vi "Lockin-4461_Multiple Inputs and Outputs_KH_functional_global_waveform_generalized_f_parallel_exec.vi"(8 "stop":bool) -> ()   [LabVIEW 2013]
uses:
  <vilib>/Analysis/baseanly.llb/Mean (DBL).vi
  <vilib>/Analysis/2dsp.llb/Decimate (single shot).vi
  <vilib>/Analysis/2dsp.llb/Decimate (single shot, DBL).vi
  DAQ-Lockin-SubVI/Lock-in Globles Multiple Inputs and Outputs used with FGV.vi
  <vilib>/Utility/error.llb/Error Cluster From Error Code.vi
  <vilib>/Analysis/NI_AALBase.lvlib
panel:
  in  "X input signal":i8(slide) scale=1.0..8.0
  in  "X Tab Control 3":enum32{"Page 1", "Page 2"}(tab)
  in  "X zero offset 2":bool
  in  "X Enum":enum16{"X and Y", "R and Theta"}(ring)
  in  "X Cluster 2":T1
  in  "X AI Block Size":dbl
  in  "X order":dbl
  in  "X AI Buffer Size":dbl
  in  "X Boolean":bool
  in  "Input Signals":i16(slide)=1 scale=1.0..20.0
  out "phase log":dbl[](array[numeric])
  in  "Tab Control 2":T2(tab)=enum."Lock-in Settings"
  in  "AI Configuration":T3(array[cluster])=[{"AI.Coupling"=10050, "AI.Max"=10.0, "AI.Min"=-10.0, "Input physical channels"="PXI1Slot2/ai0:1"}, {"AI.Coupling"=10050, "AI.Max"=10.0, "AI.Min"=-10.0, "Input physical channels"="PXI1Slot3/ai0:1"}, {"AI.Coupling"=10050, "AI.Max"=10.0, "AI.Min"=-10.0, "Input physical channels"="PXI1Slot5/ai0:1"}, {"AI.Coupling"=10050, "AI.Max"=10.0, "AI.Min"=-10.0, "Input physical channels"="PXI1Slot6/ai0:1"}] {"AI.Coupling" items=["AC"=10045, "DC"=10050, "GND"=10066]}
  in  "AO Configuration":T4(array[cluster])=[{"Output physical channels"="PXI1Slot2/ao0:1", "AO. Max"=0.1, "AO.Min"=-0.1}, {"Output physical channels"="PXI1Slot3/ao0:1", "AO. Max"=0.25, "AO.Min"=-0.25}, {"Output physical channels"="PXI1Slot5/ao0:1", "AO. Max"=0.1, "AO.Min"=-0.1}, {"Output physical channels"="PXI1Slot6/ao0:1", "AO. Max"=0.1, "AO.Min"=-0.1}]
  in  "Lockin":T5={"REF f (Hz)"=[13.0, 13.0, 13.0, 13.0, 13.0, 13.0, 13.0, 13.0], "REF phi (deg)"=[0.0, 0.0, 0.0, 0.0, 0.0, 0.0, 0.0, 0.0]} {"REF phi (deg)" format="%#_3g"}
  in  "REF f = AO f?":bool
  in  "Gain":dbl[](array[numeric])=[1.0, 1.0, 1.0, 1.0, 1.0, 1.0, 1.0, 1.0]
  out "elapsed time":dbl=1410.416
  in  "zero offset":bool
  in  "measure offset":bool
  out "filter fC (Hz)":dbl=0.3183098861837907
  in  "TC (s)":dbl=0.5
  in  "order":i32=2
  in  "AO":T6={"AO amp (V)"=[0.1, 0.09, 0.08, 0.07, 0.06, 0.05, 0.04, 0.03], "AO DC (V)"=[0.0, 0.0, 0.0, 0.0, 0.0, 0.0, 0.0, 0.0], "AO f (Hz)"=[13.0, 13.0, 13.0, 13.0, 13.0, 13.0, 13.0, 13.0], "AO phi (deg)"=[0.0, 0.0, 0.0, 0.0, 0.0, 0.0, 0.0, 0.0], "function"=[enum."Sine Wave", enum."Sine Wave", enum."Sine Wave", enum."Sine Wave", enum."Sine Wave", enum."Sine Wave", enum."Sine Wave", enum."Sine Wave"]} {"AO DC (V)" format="%#_6p"; "AO amp (V)" format="%#_6p"}
  in  "all  f same?":bool
  in  "simulate?":bool=TRUE
  in  "reset signal":bool
  in  "AI Buffer Size (S)":i32=10
  in  "milliseconds to wait":u32=1000
  out "sampling info":cluster{"Fs":dbl, "#s":dbl}={"Fs"=204800.0, "#s"=15753.0}
  in  "pre filter fl":dbl=40.0
  in  "prefilter?":bool
  in  "reset REF phi to zero":bool
  in  "autophase?":bool
  in  "auto block size":bool=TRUE
  in  "P":dbl=0.5 format="%.2f"
  in  "I":dbl=0.6 format="%.2f"
  in  "D":dbl=0.019999999999999997 format="%.2f"
  out "Display 2":dbl=-0.01728566342801391 format="%.6p"
  out "Display 1":dbl=0.09985345527594 format="%.6p"
  in  "Display":enum16{"X and Y", "R and Theta"}(ring)=enum."R and Theta"
  out "AO Task":refnum<k21>[](array[refnum])
  out "AI task":refnum<k21>[](array[refnum])
  in  "Tab Control":T7(tab)
  out "Display X (or R)":waveform(dbl)[](graph)=[{"t0"=timestamp(3507304728.547973 s since 1904-01-01), "dt"=1.0, "Y"=[0.09985345527594]}, {"t0"=timestamp(3507304728.547973 s since 1904-01-01), "dt"=1.0, "Y"=[0.090216464470275]}, {"t0"=timestamp(3507304728.547973 s since 1904-01-01), "dt"=1.0, "Y"=[0.07984767344892373]}, {"t0"=timestamp(3507304728.547973 s since 1904-01-01), "dt"=1.0, "Y"=[0.06948646282319876]}, {"t0"=timestamp(3507304728.547973 s since 1904-01-01), "dt"=1.0, "Y"=[0.0610513314084819]}, {"t0"=timestamp(3507304728.547973 s since 1904-01-01), "dt"=1.0, "Y"=[0.0501207617290639]}, {"t0"=timestamp(3507304728.547973 s since 1904-01-01), "dt"=1.0, "Y"=[0.04039608724889331]}, {"t0"=timestamp(3507304728.547973 s since 1904-01-01), "dt"=1.0, "Y"=[0.029866562813137317]}]
  out "Display Y (or Theta)":waveform(dbl)[](graph)=[{"t0"=timestamp(3507304728.547973 s since 1904-01-01), "dt"=1.0, "Y"=[-0.01728566342801391]}, {"t0"=timestamp(3507304728.547973 s since 1904-01-01), "dt"=1.0, "Y"=[-0.32961665980326604]}, {"t0"=timestamp(3507304728.547973 s since 1904-01-01), "dt"=1.0, "Y"=[-0.26399334892304605]}, {"t0"=timestamp(3507304728.547973 s since 1904-01-01), "dt"=1.0, "Y"=[-0.3359989409283301]}, {"t0"=timestamp(3507304728.547973 s since 1904-01-01), "dt"=1.0, "Y"=[0.18728664235110717]}, {"t0"=timestamp(3507304728.547973 s since 1904-01-01), "dt"=1.0, "Y"=[0.053789543137479]}, {"t0"=timestamp(3507304728.547973 s since 1904-01-01), "dt"=1.0, "Y"=[0.07133775541983144]}, {"t0"=timestamp(3507304728.547973 s since 1904-01-01), "dt"=1.0, "Y"=[-0.34211850150716916]}]
  in  "\"master\" lockin channel":i32
  out "Waveform Graph":waveform(dbl)[](graph)
  in  "decimating factor":i32=1
  out "Results (X, Y, R, Theta)":dbl[][](array[numeric])=[[0.09985345073171382, -3.0124962231235766e-05, 0.09985345527594, -0.01728566342801391], [0.09021497158081004, -0.0005190030732351189, 0.090216464470275, -0.32961665980326604], [0.07984682588549666, -0.0003679010969547394, 0.07984767344892373, -0.26399334892304605], [0.0694852680113616, -0.00040748628079075754, 0.06948646282319876, -0.3359989409283301], [0.06105100524667845, 0.0001995623169072153, 0.0610513314084819, 0.18728664235110717], [0.050120739641995225, 4.705359630329193e-05, 0.0501207617290639, 0.053789543137479], [0.04039605593746594, 5.029629532938592e-05, 0.04039608724889331, 0.07133775541983144], [0.02986603038399768, -0.0001783350027455678, 0.029866562813137317, -0.34211850150716916]] format="%#_6p"
  out "offsets":dbl[](array[numeric])
  # "SIMPLIFY THIS !!!!!!!!!!!!!!!!!!!!!!!!!!!!!!!!!!!!!!!!!!!!!!!!!!!!!!!!!!"
  # "Real time Adjustable Values"
  # "WAVEFORM 2"
  # "Configurations"
  # "should this be x multiple\nof the frequency?"
  # "Features:\n1, Any number of input and output channels\n2, Each AO outputs an DC+AC signal, DC for sample biasing and AC for OSC. These values can be adjusted in real time.\n3, Synchronous filtering\n\nInstructions:\n1, Array index of AI configuration and AO configuration refers to task.\n2, Array index in Amplifier Settings, Phase$&Tc control , and gains correlates to channel number.\n3, Each 4461 board can have 2 lock-in channels. Syntax for 2 channles, e.g. PXI1Slot2/ai0:1. If you want to use just one, then PXI1Slot2/ai0.\n4, Parameters (especially DC value for sample biasing) can be remotely controlled by clicking \"local\"and \"remote\" button. In real experiments, put golable values (can be found in Lock-in globles.vi) in your VI to control the lock-in and read out.\n5, choose OSC frequencies to be multiple of \nAI Rate/AI Block SIze to have best performance.\n\n-Guanglei 06/23/2011\n\nUpdate:\n1. Allows any number of lockin amplifiers and AO tasks.\n2. Delete the channels from any AI/AO Configuration elements you do not want to use.\n3. Rows (first index) of the OSC Configuration correspond to different AO tasks, while columns (second index) correspond to AO channels in that task. All channels in a given element of the AO Configuration array will go into a single task.\n4. The same number of output channels must go in each AO task.\n5. Make sure a Phase&Tc element and an Amplifier Settings element is set for each AI channel.\n-Joe 12/3/2013"
  # "signal\n*sine\n*cosine\n*2\n*2\nLP filter\nLP filter"
  # "auto decimate so total # points is certain value? (O 1000?)"
  # "hide stuff here in this tab"
  # "multiple of frequency??"
  # "this is \"time constant\""
  # "The top array index selects which card you are setting the outputs for,and the second index selects which output chanel on that card.\n\nFor Phase&Tc, you must have an array element initialized for each input signal."
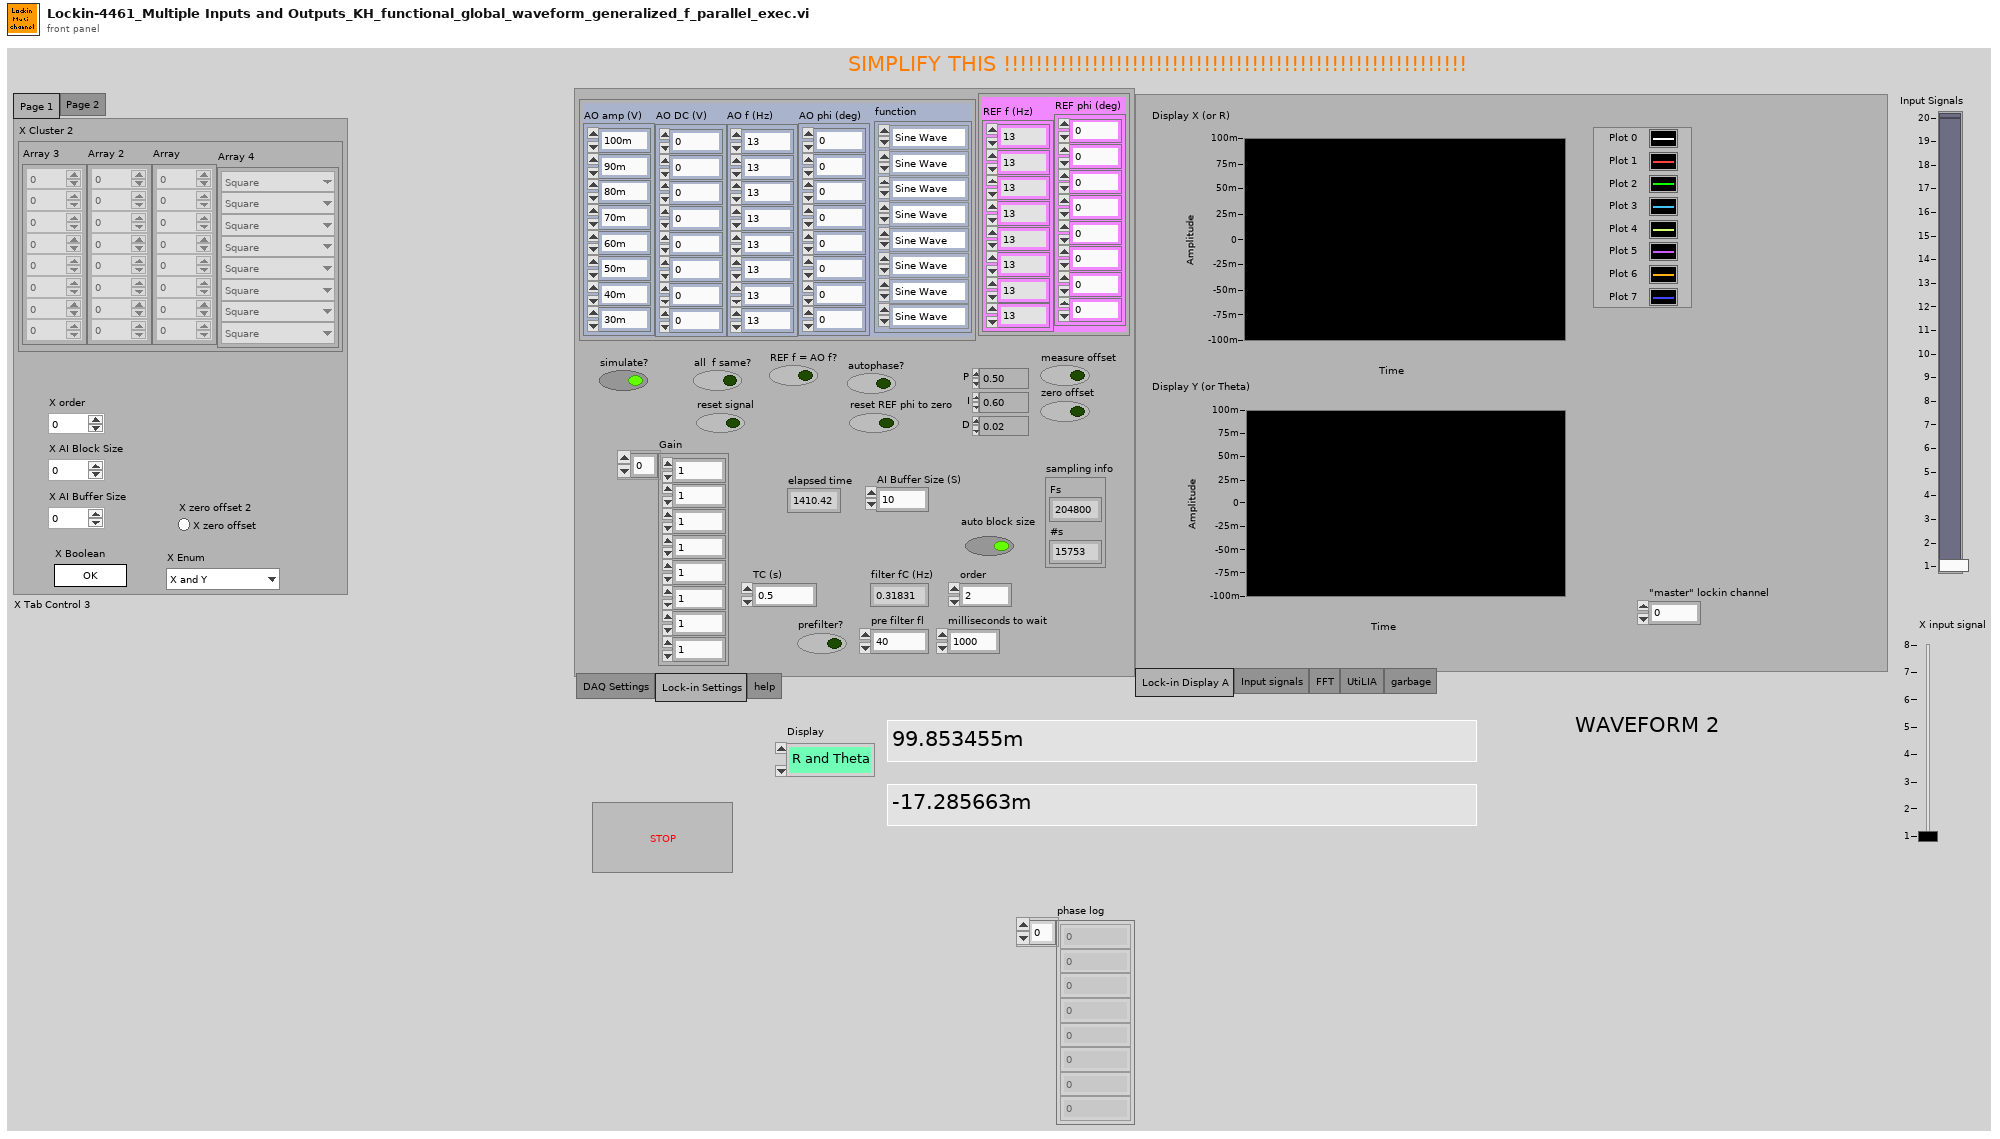
[diagram p1: front panel]
types:
  T1 = cluster{"Array":dbl[], "Array 2":dbl[], "Array 3":dbl[], "Array 4":enum16{"Square\n", "Sine", "Triangle"}[]}
  T2 = enum32{"DAQ Settings", "Lock-in Settings", "help"}
  T3 = cluster{"AI.Coupling":i32, "AI.Max":dbl, "AI.Min":dbl, "Input physical channels":tag}[]
  T4 = cluster{"Output physical channels":tag, "AO. Max":dbl, "AO.Min":dbl}[]
  T5 = cluster{"REF f (Hz)":dbl[], "REF phi (deg)":dbl[]}
  T6 = cluster{"AO amp (V)":dbl[], "AO DC (V)":dbl[], "AO f (Hz)":dbl[], "AO phi (deg)":dbl[], "function":enum16{"Sine Wave", "Triangle Wave", "Square Wave", "Sawtooth Wave"}[]}
  T7 = enum32{"Lock-in Display A", "Input signals", "FFT", "UtiLIA", "garbage"}
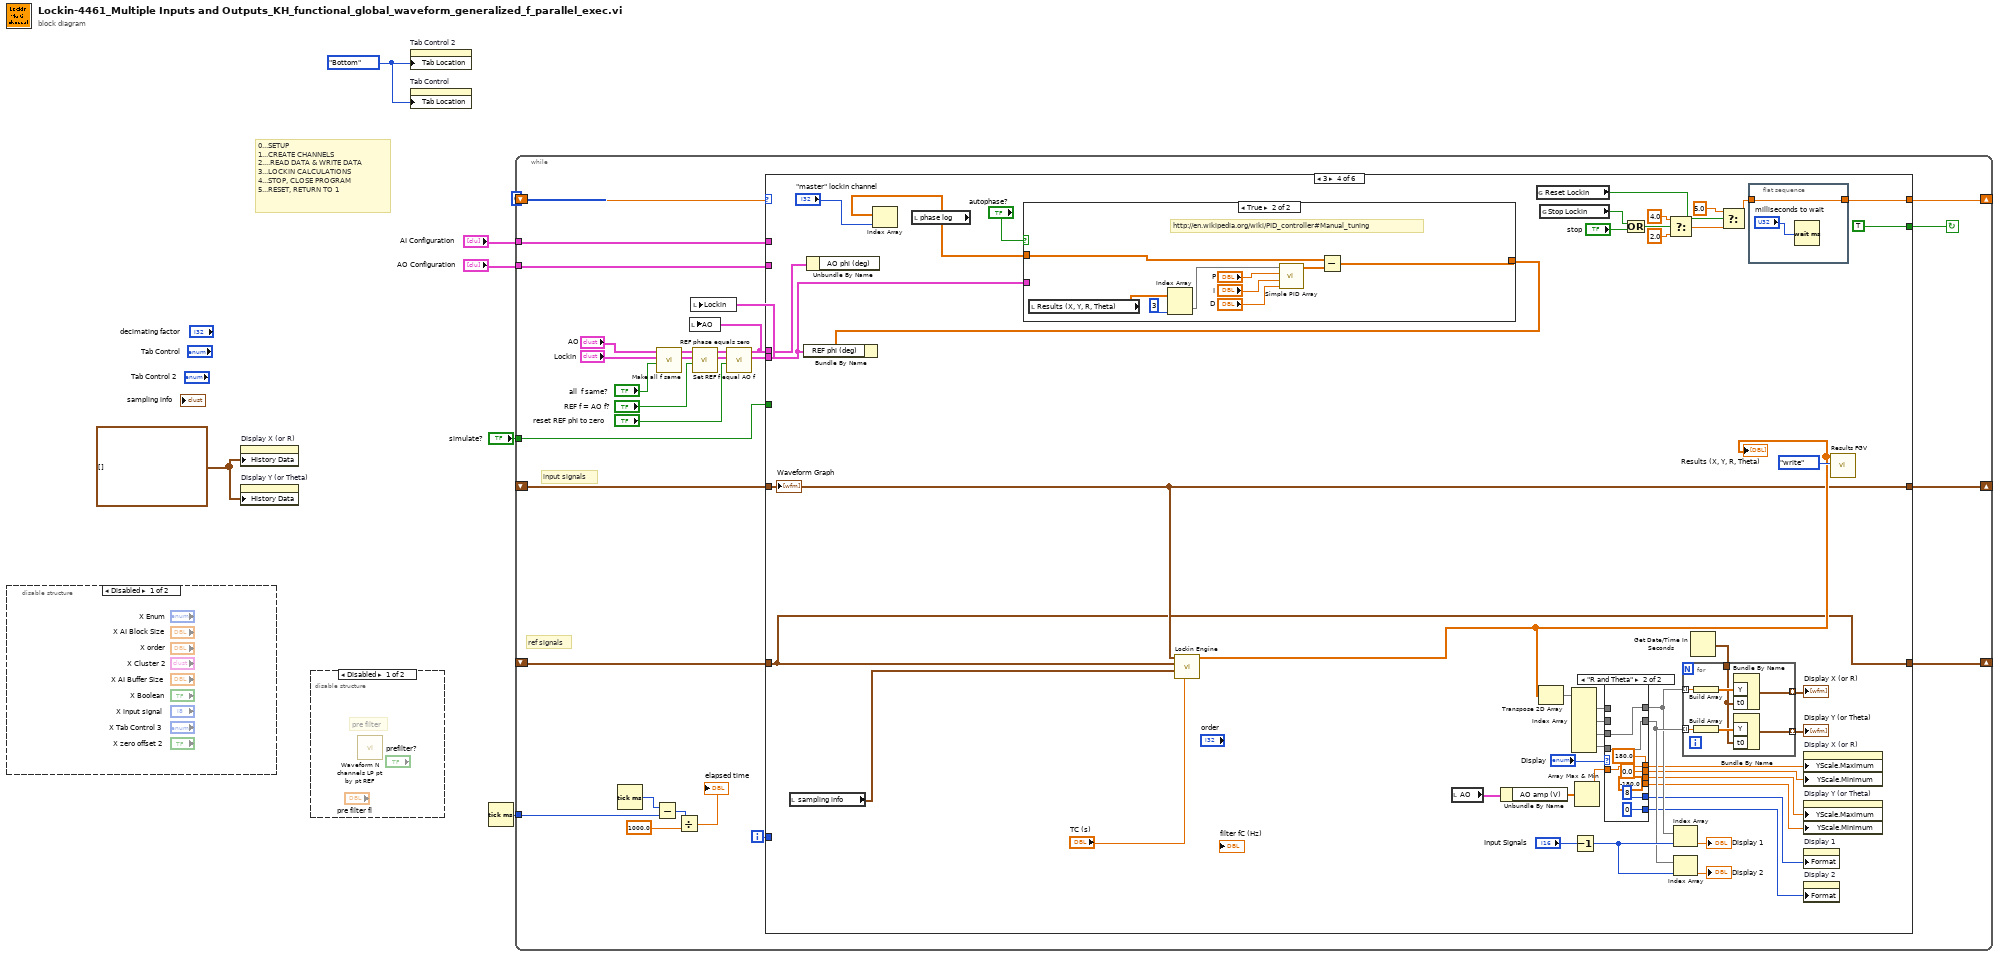
[diagram p0: block diagram]
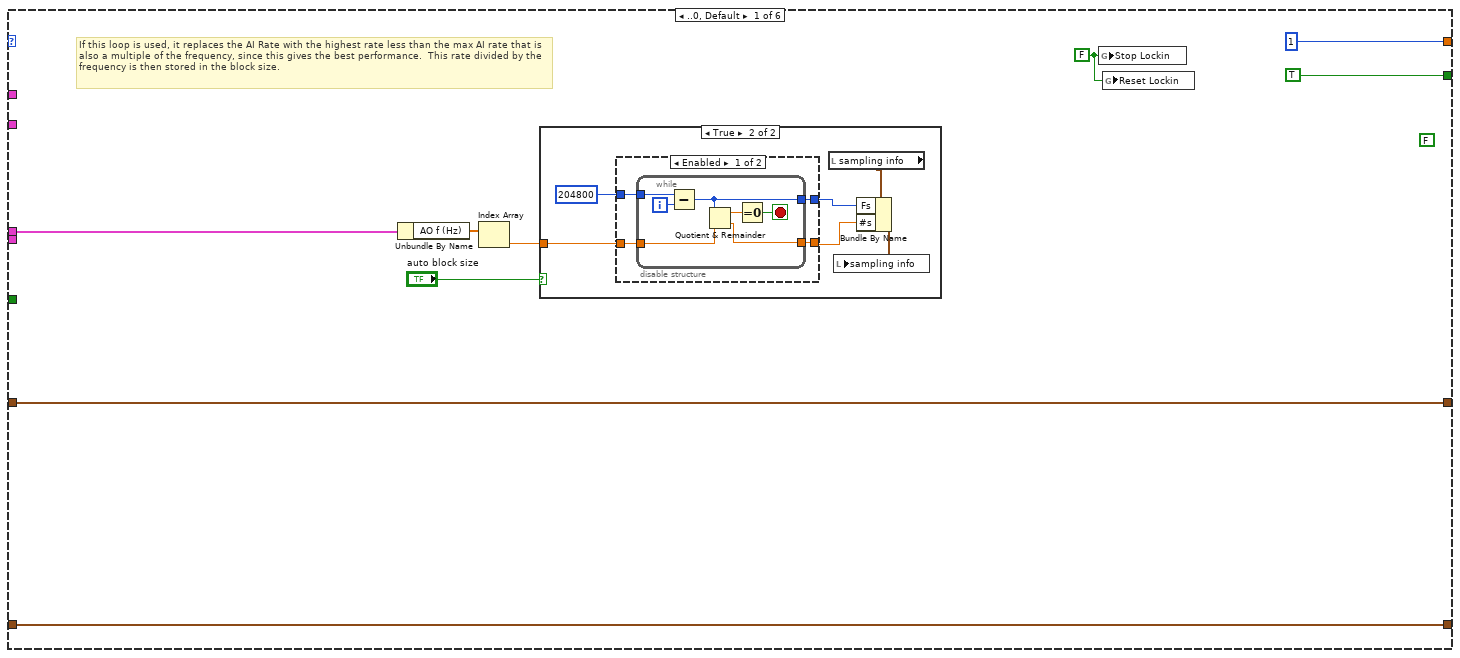
[diagram p4: hidden frame]
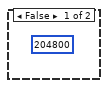
[diagram p5: hidden frame]
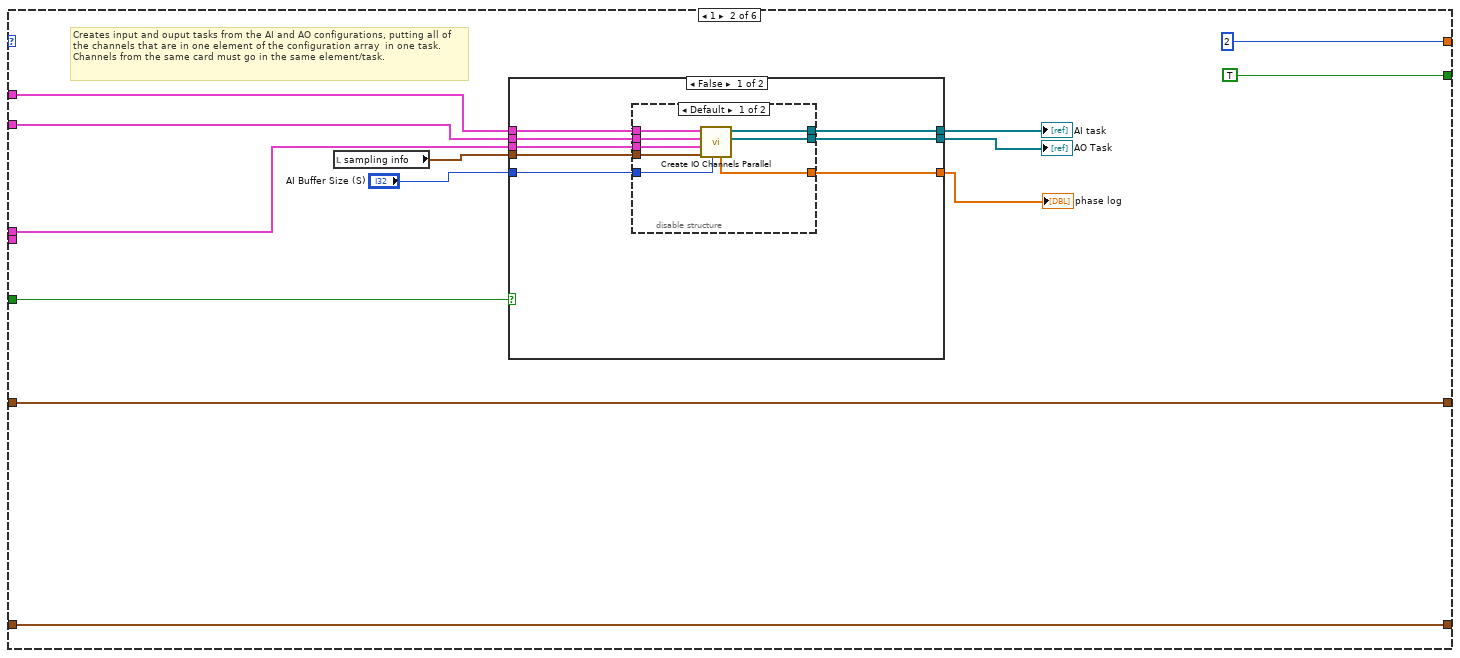
[diagram p7: hidden frame]
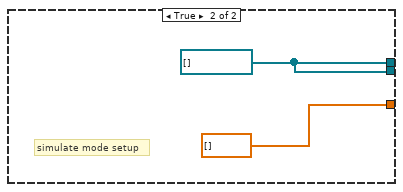
[diagram p9: hidden frame]
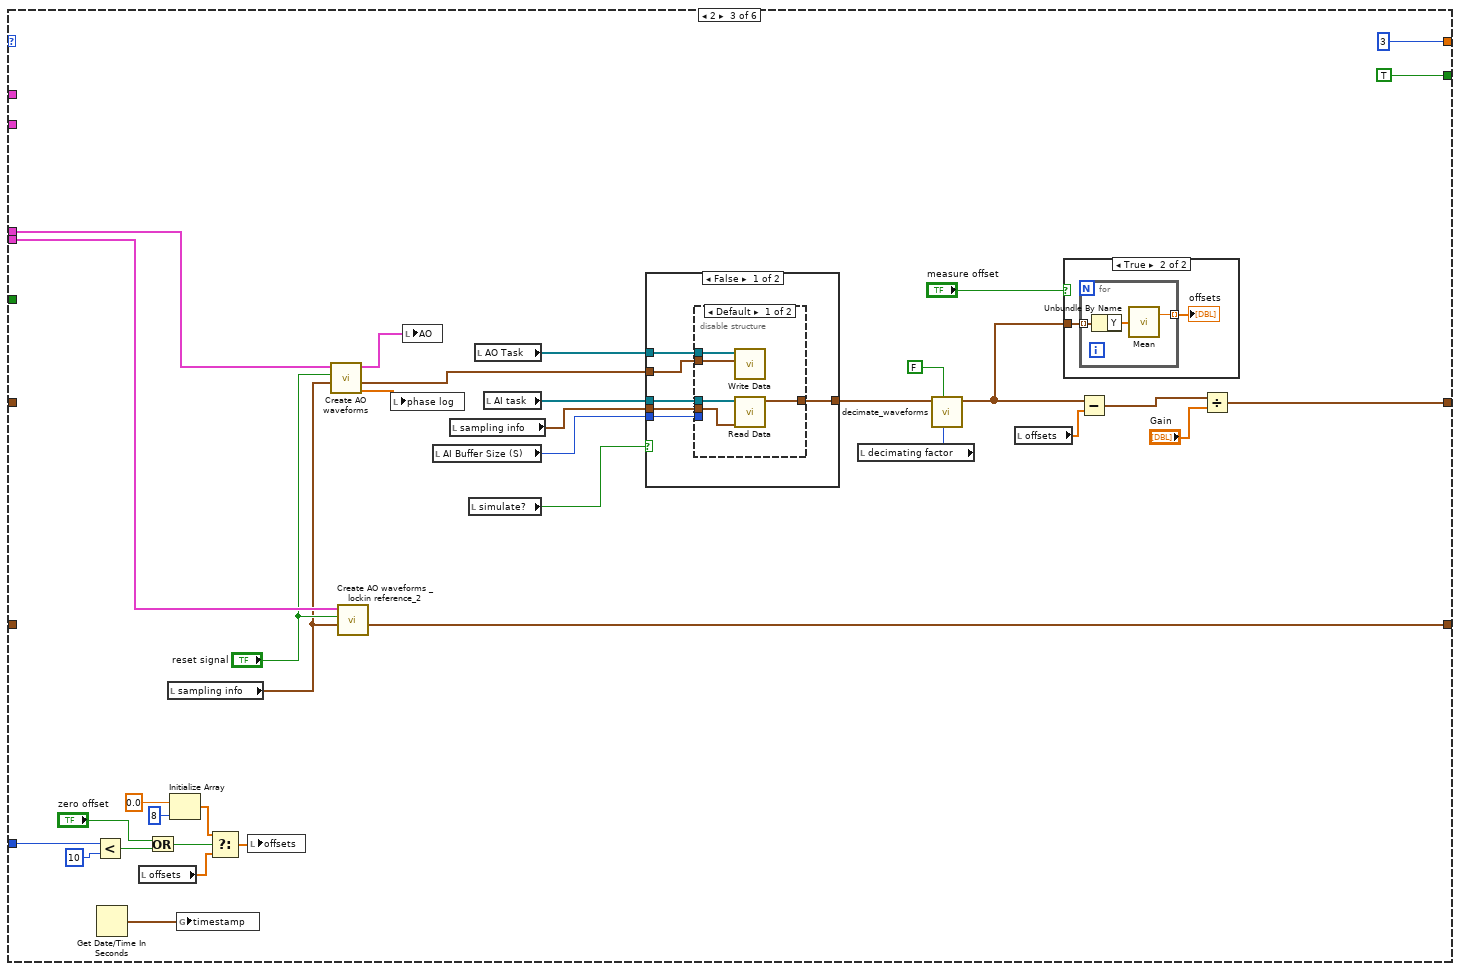
[diagram p10: hidden frame]
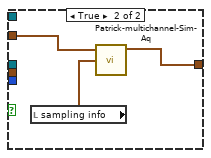
[diagram p12: hidden frame]
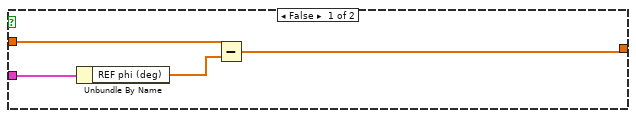
[diagram p14: hidden frame]
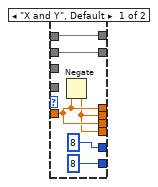
[diagram p15: hidden frame]
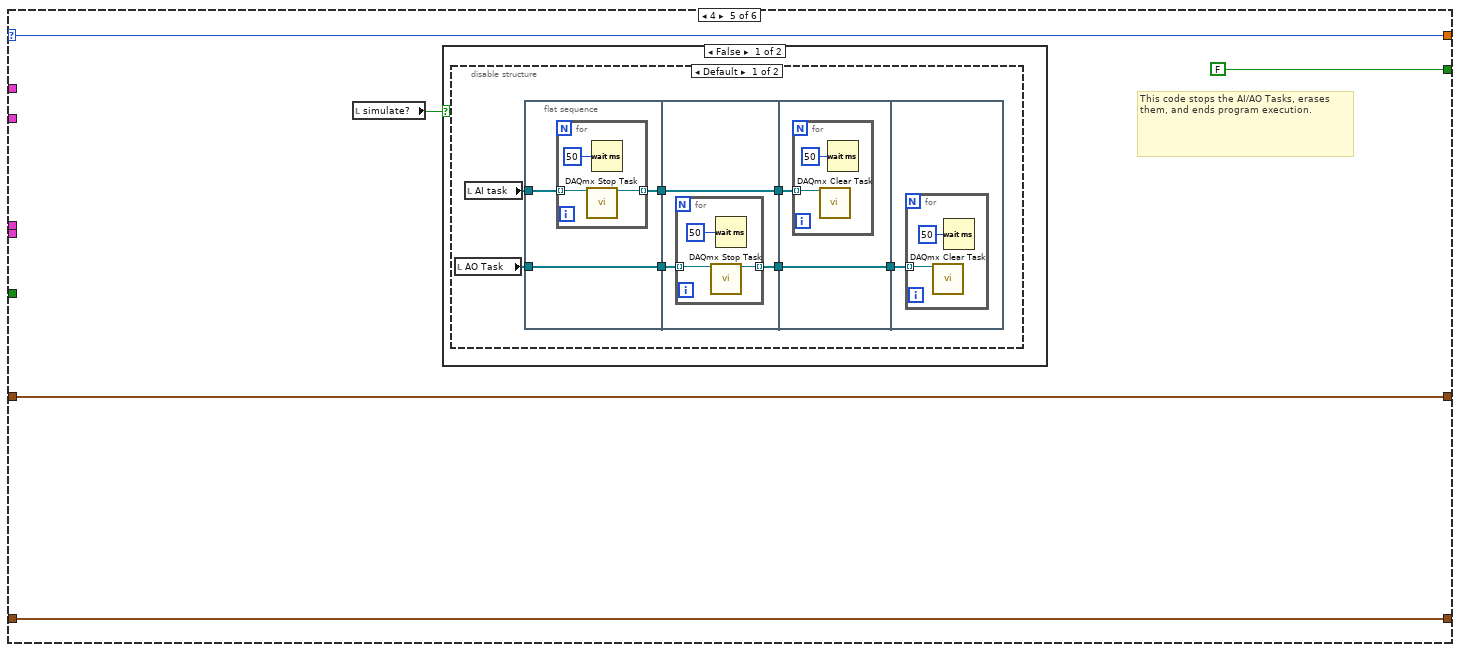
[diagram p16: hidden frame]
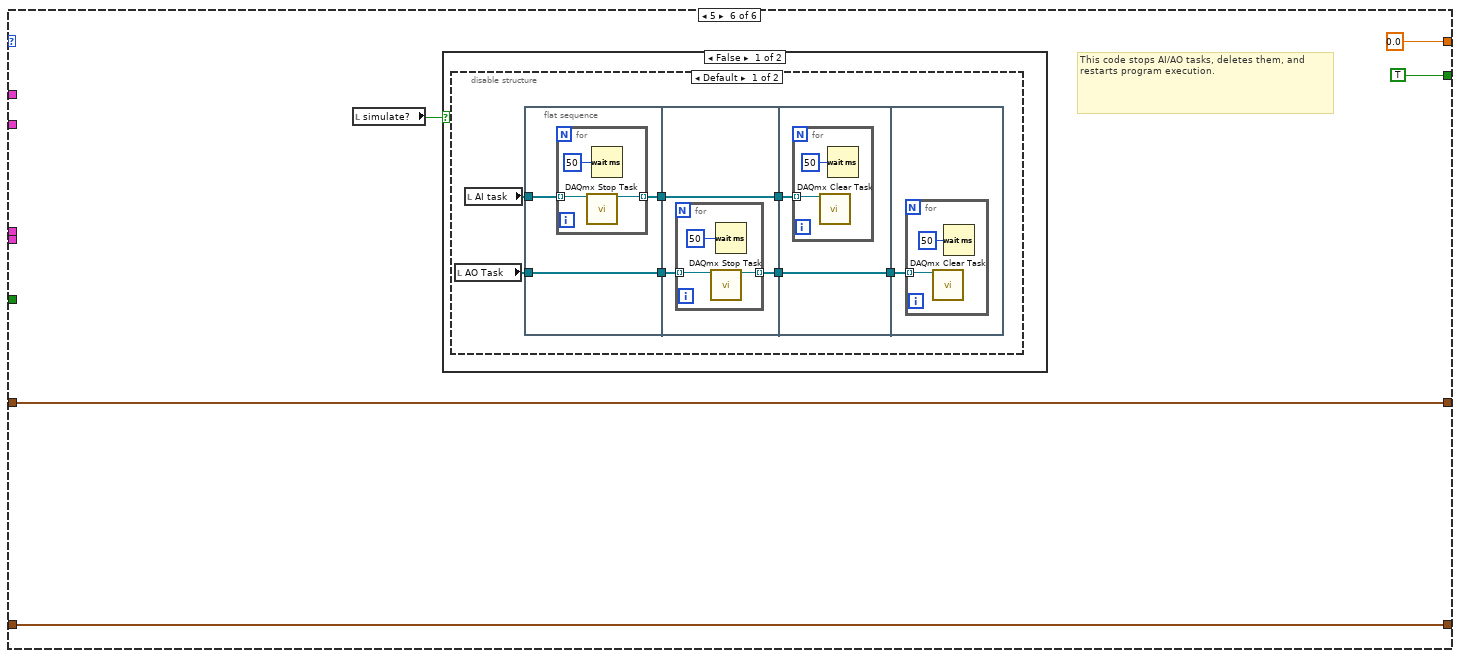
[diagram p19: hidden frame]
diagram:
  w2 = waveform(dbl)[][] [] ("History Data")
  w1 = enum32{"Top", "Bottom", "Left", "Right"}."Bottom" ("Tab Location")
  # "0...SETUP\n1...CREATE CHANNELS\n2....READ DATA & WRITE DATA\n3...LOCKIN CALCULATIONS\n4...STOP, CLOSE PROGRAM\n5...RESET, RETURN TO 1"
  n1 = disable-structure shown="Disabled" {
    frame Disabled {
    }
    frame Enabled {
    }
  }
  n2 = property on="Display X (or R)" class="WaveformChart (strict)"("History Data"=w2) -> ()  [unwired: 2 in, 2 out]
  n3 = property on="Display Y (or Theta)" class="WaveformChart (strict)"("History Data"=w2) -> ()  [unwired: 2 in, 2 out]
  n4 = disable-structure shown="Disabled" {
    frame Disabled {
      # "pre filter"
      n5 = call "Waveform N channels LP pt by pt REF.vi"() -> ()  [unwired: 11 in, 1 out]
    }
    frame Enabled {
    }
  }
  n6 = property on="Tab Control 2" class="TabCtl (strict)"("Tab Location"=w1) -> ()  [unwired: 2 in, 2 out]
  n7 = property on="Tab Control" class="TabCtl (strict)"("Tab Location"=w1) -> ()  [unwired: 2 in, 2 out]
  n8 = Tick Count (ms)() -> (millisecond timer value=w6:u32)
  n9 = while {
    shift-right: [w34] -> _
    shift-left: 0 -> [w33]
    tunnel: "AI Configuration" -> [w32]
    tunnel: "AO Configuration" -> [w31]
    shift-right: [w30] -> _
    shift-left: _ -> [w29]
    tunnel: w6 -> [w28]
    tunnel: "simulate?" -> [w9]
    shift-right: [w12] -> _
    shift-left: _ -> [w8]
    i -> [w25]
    stop <- w26 continue-if-true
    # "ref signals"
    # "input signals"
    n10 = Tick Count (ms)() -> (millisecond timer value=w24:u32)
    n11 = Subtract(x=w24, y=w28) -> (x-y=w27:u32)
    n12 = call "Make all f same.vi"("all  frequencies same?"="all  f same?", "Lockin"="Lockin", "AO"="AO") -> ("Lockin 2"=w21:T5, "AO 2"=w22:T6)  [unwired: 7 in]
    n13 = Divide(x=w27, y=1000.0) -> (x/y=→"elapsed time":dbl)
    n14 = call "Set REF f equal AO f.vi"("REE = AO?"="REF f = AO f?", "Lockin"=w21, "AO"=w22) -> ("Lockin 2"=w20:T5, "AO 2"=w18:T6)  [unwired: 7 in]
    n15 = call "REF phase equals zero.vi"("reset REF phi to zero"="reset REF phi to zero", "Lockin"=w20, "AO"=w18) -> ("Lockin 2"=w15:T5, "AO 2"=w14:T6)  [unwired: 7 in]
    n16 = local write "AO"(w14) -> ()
    n17 = local write "Lockin"(w15) -> ()
    n18 = case shown="3" w33 {
      selector: w33 -> [_ _ _ _ w234 _]
      tunnel: [1 2 3 w177 w234 0.0 ("f")] -> w34
      tunnel: w32 -> [_ w65 _ _ _ _]
      tunnel: [TRUE TRUE TRUE TRUE FALSE TRUE] -> w26
      tunnel: w31 -> [_ w66 _ _ _ _]
      tunnel: [w39 w72 w109 w150 w233 w264] -> w30
      tunnel: w29 -> [w39 w72 _ w150 w233 w264]
      tunnel: w25 -> [_ _ w122 _ _ _]
      tunnel: w9 -> [_ w69 _ _ _ _]
      tunnel: w14 -> [w38 w67 w101 w154 _ _]
      tunnel: w15 -> [_ _ w100 w156 _ _]
      tunnel: [w35 w64 w94 w148 w231 w262] -> w12
      tunnel: w8 -> [w35 w64 _ w148 w231 w262]
      frame ..0, Default {
        (unwired) FALSE ("reset signal?")
        w42 = FALSE ("Stop Lockin")
        # "If this loop is used, it replaces the AI Rate with the highest rate less than the max AI rate that is also a multiple of the frequency, since this gives the best performance.  This rate divided by the frequency is then stored in the block size."
        n19 = Unbundle By Name(w38) -> ("AO f (Hz)"=w37:dbl[])
        n20 = Index Array(array=w37) -> (element=w36:dbl)  [unwired: 1 in]
        n21 = case shown="True" "auto block size" {
          tunnel: w36 -> [_ w48]
          frame False {
            (unwired) 204800 ("max ai rate")
          }
          frame True {
            n22 = disable-structure shown="Enabled" {
              disable-tunnel: [w53 w61] -> w45
              disable-tunnel: [w52 w62] -> w46
              disable-tunnel: 204800 ("max ai rate") -> [w51 w62]
              disable-tunnel: w48 -> [w50 w61]
              frame Enabled {
                n23 = while {
                  tunnel: w51 -> [w60]
                  tunnel: [w58] -> w53
                  tunnel: [w56] -> w52
                  tunnel: w50 -> [w57]
                  i -> [w59]
                  stop <- w54 stop-if-true
                  n24 = Subtract(x=w60, y=w59) -> (x-y=w56:i32)
                  n25 = Quotient & Remainder(x=w56, y=w57) -> (x-y*floor(x/y)=w55:dbl, floor(x/y)=w58:dbl)
                  n26 = Equal To 0?(x=w55) -> (x = 0?=w54:bool)
                }
              }
              frame Disabled {
              }
            }
            n27 = local read "sampling info"() -> (w47:cluster{"Fs":dbl, "#s":dbl})
            n28 = Bundle By Name(cluster=w47, "Fs"=w46, "#s"=w45) -> (w44:cluster{"Fs":dbl, "#s":dbl})
            n29 = local write "sampling info"(w44) -> ()
          }
        }
        n30 = global write "Lock-in Globles Multiple Inputs and Outputs used with FGV.vi" "Stop Lockin"(w42) -> ()
        n31 = global write "Lock-in Globles Multiple Inputs and Outputs used with FGV.vi" "Reset Lockin"(w42) -> ()
      }
      frame 1 {
        # "Creates input and ouput tasks from the AI and AO configurations, putting all of the channels that are in one element of the configuration array  in one task.  Channels from the same card must go in the same element/task."
        n32 = local read "sampling info"() -> (w63:cluster{"Fs":dbl, "#s":dbl})
        n33 = case shown="False" w69 {
          tunnel: w65 -> [w83 _]
          tunnel: w66 -> [w82 _]
          tunnel: [w81 w93] -> w73
          tunnel: w63 -> [w80 _]
          tunnel: [w79 w93] -> w71
          tunnel: "AI Buffer Size (S)" -> [w78 _]
          tunnel: [w77 dbl[] [] ("phase log")] -> w70
          tunnel: w67 -> [w76 _]
          frame False {
            n34 = disable-structure shown="Default" {
              disable-tunnel: w83 -> [w91 _]
              disable-tunnel: w82 -> [w90 _]
              disable-tunnel: [w89 _] -> w81
              disable-tunnel: w80 -> [w85 _]
              disable-tunnel: [w88 _] -> w79
              disable-tunnel: w78 -> [w87 _]
              disable-tunnel: [w86 _] -> w77
              disable-tunnel: w76 -> [w84 _]
              frame condition #0 (active) {
                n35 = call "Create IO Channels Parallel.vi"("AI Buffer Size (s)"=w87, "sampling info"=w85, "AO"=w84, "AO Configuration"=w90, "AI Configuration"=w91) -> ("AO Task"=w88:refnum<k21>[], "AI task"=w89:refnum<k21>[], "phase log"=w86:dbl[])  [unwired: 3 in, 1 out]
              }
              frame condition #1 {
              }
            }
          }
          frame True {
            w93 = refnum<k21>[] [] ("AI task")
            # "simulate mode setup"
          }
        }
        "AO Task" <- w71
        "AI task" <- w73
        "phase log" <- w70
      }
      frame 2 {
        n36 = Less?(x=w122, y=10) -> (x < y?=w115:bool)
        n37 = Get Date/Time In Seconds() -> (seconds since 1Jan1904=w126:timestamp)
        n38 = local read "offsets"() -> (w121:dbl[])
        n39 = Or(x="zero offset", y=w115) -> (x .or. y?=w114:bool)
        n40 = local read "sampling info"() -> (w98:cluster{"Fs":dbl, "#s":dbl})
        n41 = Initialize Array(0.0, 8 ("dimension size")) -> (w118:dbl[])
        n42 = global write "Lock-in Globles Multiple Inputs and Outputs used with FGV.vi" "timestamp"(w126) -> ()
        n43 = Select(t=w118, s=w114, f=w121) -> (s? t:f=w120:dbl[])
        n44 = local write "offsets"(w120) -> ()
        n45 = call "Create AO waveforms.vi"("sampling info"=w98, "reset signal"="reset signal", "AO"=w101) -> ("phase out"=w97:dbl[], "AO Array"=w96:waveform(dbl)[], "AO 2"=w95:T6)  [unwired: 6 in]
        n46 = call "Create AO waveforms _lockin reference_2.vi"("sampling info"=w98, "reset signal"="reset signal", "Lockin"=w100) -> ("AO Array"=w94:waveform(dbl)[])  [unwired: 6 in, 2 out]
        n47 = local write "phase log"(w97) -> ()
        n48 = local write "AO"(w95) -> ()
        n49 = local read "AI Buffer Size (S)"() -> (w124:i32)
        n50 = local read "sampling info"() -> (w125:cluster{"Fs":dbl, "#s":dbl})
        n51 = local read "simulate?"() -> (w108:bool)
        n52 = local read "AO Task"() -> (w105:refnum<k21>[])
        n53 = local read "AI task"() -> (w110:refnum<k21>[])
        n54 = case shown="False" w108 {
          tunnel: w110 -> [w134 _]
          tunnel: w125 -> [w133 _]
          tunnel: w124 -> [w132 _]
          tunnel: [w130 w142] -> w107
          tunnel: w96 -> [w129 w140]
          tunnel: w105 -> [w131 _]
          frame False {
            n55 = disable-structure shown="Default" {
              disable-tunnel: w134 -> [w139 _]
              disable-tunnel: w133 -> [w135 _]
              disable-tunnel: w132 -> [_ _]
              disable-tunnel: [w138 _] -> w130
              disable-tunnel: w131 -> [w137 _]
              disable-tunnel: w129 -> [w136 _]
              frame condition #0 (active) {
                n56 = call "Write Data.vi"("AO Array"=w136, "AO Task"=w137) -> ()  [unwired: 10 in]
                n57 = call "Read Data.vi"("sampling info"=w135, "AI task"=w139) -> ("Input Signals"=w138:waveform(dbl)[])  [unwired: 7 in, 2 out]
              }
              frame condition #1 {
              }
            }
          }
          frame True {
            n58 = local read "sampling info"() -> (w141:cluster{"Fs":dbl, "#s":dbl})
            n59 = call "Patrick-multichannel-Sim-Aq.vi"("data"=w140, "sampling info"=w141) -> ("Data"=w142:waveform(dbl)[])  [unwired: 5 in]
          }
        }
        n60 = local read "decimating factor"() -> (w104:i32)
        n61 = call "decimate_waveforms.vi"("decimating factor"=w104, "averaging"=FALSE, "Input Signal"=w107) -> ("Decimated Waveforms"=w112:waveform(dbl)[])  [unwired: 7 in, 1 out]
        n62 = local read "offsets"() -> (w102:dbl[])
        n63 = case shown="True" "measure offset" {
          tunnel: w112 -> [_ w143]
          frame False {
          }
          frame True {
            n64 = for {
              tunnel: [w147] -> w144 mode=indexing
              tunnel: w143 -> [w146] mode=indexing
              n65 = Unbundle By Name(w146) -> ("Y"=w145:dbl[])
              n66 = call-poly <vilib>:"Mean.vi"("X"=w145) -> ("mean"=w147:dbl)  [unwired: 1 out]
            }
            "offsets" <- w144
          }
        }
        n67 = Subtract(x=w112, y=w102) -> (x-y=w111:waveform(dbl)[])
        n68 = Divide(x=w111, y="Gain") -> (x/y=w109:waveform(dbl)[])
      }
      frame 3 {
        n69 = local read "sampling info"() -> (w149:cluster{"Fs":dbl, "#s":dbl})
        n70 = Unbundle By Name(w154) -> ()  [unwired: 1 out]
        n71 = local read "phase log"() -> (w151:dbl[])
        n72 = Index Array(array=w151, index="\"master\" lockin channel") -> ()  [unwired: 1 out]
        n73 = case shown="True" "autophase?" {
          tunnel: [w198 w207] -> w155
          tunnel: w156 -> [w197 _]
          tunnel: w151 -> [w195 w199]
          frame False {
            n74 = Unbundle By Name(w197) -> ("REF phi (deg)"=w196:dbl[])
            n75 = Subtract(x=w195, y=w196) -> (x-y=w198:dbl[])
          }
          frame True {
            # "http://en.wikipedia.org/wiki/PID_controller#Manual_tuning"
            n76 = local read "Results (X, Y, R, Theta)"() -> (w205:dbl[][])
            n77 = Index Array(array=w205, index (col)=3 ("index (row)")) -> (element=w204:dbl[])  [unwired: 1 in]
            n78 = call "Simple PID Array.vi"("D"="D", "I"="I", "P"="P", "process variable"=w204) -> ("output value"=w200:dbl[])  [unwired: 7 in]
            n79 = Subtract(x=w199, y=w200) -> (x-y=w207:dbl[])
          }
        }
        n80 = Bundle By Name(cluster=w156, "REF phi (deg)"=w155) -> ()  [unwired: 1 out]
        n81 = call "Lockin Engine.vi"("TC (s)"="TC (s)", "sampling info"=w149, "Reference In"=w148, "Signal in"=w150) -> ("Results (X,Y,R,Theta)"=w179:dbl[][])  [unwired: 6 in, 1 out]
        "Results (X, Y, R, Theta)" <- w179
        n82 = local read "AO"() -> (w162:T6)
        n83 = Unbundle By Name(w162) -> ("AO amp (V)"=w161:dbl[])
        n84 = global read "Lock-in Globles Multiple Inputs and Outputs used with FGV.vi" "Reset Lockin"() -> (w186:bool)
        n85 = Transpose 2D Array(2D array=w179) -> (transposed array=w180:dbl[][])
        n86 = global read "Lock-in Globles Multiple Inputs and Outputs used with FGV.vi" "Stop Lockin"() -> (w192:bool)
        n87 = Index Array(array=w180) -> (element #1=w183:dbl[], element #2=w182:dbl[], element #3=w181:dbl[], element #4=w172:dbl[])  [unwired: 8 in]
        n88 = Decrement(x="Input Signals") -> (x-1=w170:i16)
        n89 = Array Max & Min(array=w161) -> (max value=w160:dbl)  [unwired: 3 out]
        n90 = case shown="\"R and Theta\"" "Display" {
          tunnel: w183 -> [w221 _]
          tunnel: [w221 w230] -> w166
          tunnel: w182 -> [w222 _]
          tunnel: [w222 w229] -> w167
          tunnel: w181 -> [_ w230]
          tunnel: w172 -> [_ w229]
          tunnel: [u8 8 ("Display Format:Format") u8 0 ("Display Format:Format")] -> w164
          tunnel: [u8 8 ("Display Format:Format") u8 8 ("Display Format:Format")] -> w163
          tunnel: w160 -> [w218 w226]
          tunnel: [w218 w226] -> w159
          tunnel: [w218 180.0] -> w158
          tunnel: [w217 0.0] -> w152
          tunnel: [w217 -180.0] -> w157
          frame "X and Y", Default {
            n91 = Negate(x=w218) -> (-x=w217:dbl)
          }
          frame "R and Theta" {
          }
        }
        n92 = Or(x=w192, y="stop") -> (x .or. y?=w190:bool)
        n93 = Select(t=4.0 ("f"), s=w190, f=2.0) -> (s? t:f=w189:dbl)
        n94 = Index Array(array=w166, index=w170) -> (element=→"Display 1":dbl)
        n95 = Index Array(array=w167, index=w170) -> (element=→"Display 2":dbl)
        n96 = Get Date/Time In Seconds() -> (seconds since 1Jan1904=w173:timestamp)
        n97 = for {
          tunnel: w166 -> [w214] mode=indexing
          tunnel: w167 -> [w213] mode=indexing
          tunnel: [w212] -> w175 mode=indexing
          tunnel: [w211] -> w174 mode=indexing
          tunnel: w173 -> [w208]
          n98 = Build Array(w214) -> (w210:dbl[])
          n99 = Build Array(w213) -> (w209:dbl[])
          n100 = Bundle By Name("Y"=w210, "t0"=w208) -> (w212:waveform(dbl))  [unwired: 1 in]
          n101 = Bundle By Name("Y"=w209, "t0"=w208) -> (w211:waveform(dbl))  [unwired: 1 in]
        }
        "Display Y (or Theta)" <- w174
        "Display X (or R)" <- w175
        n102 = Select(t=5.0, s=w186, f=w189) -> (s? t:f=w176:dbl)
        n103 = flat-sequence {
          tunnel: [w216] -> w177
          tunnel: w176 -> [w216]
          frame #0 {
            n104 = Wait (ms)(milliseconds to wait="milliseconds to wait") -> ()  [unwired: 1 out]
          }
        }
        n105 = property on="Display X (or R)" class="WFChart (strict)"("YScale.Maximum"=w159, "YScale.Minimum"=w152) -> ()  [unwired: 2 in, 2 out]
        n106 = property on="Display Y (or Theta)" class="WFChart (strict)"("YScale.Maximum"=w158, "YScale.Minimum"=w157) -> ()  [unwired: 2 in, 2 out]
        n107 = property on="Display 1" class="DigNum (strict)"("Format"=w163) -> ()  [unwired: 2 in, 2 out]
        n108 = property on="Display 2" class="DigNum (strict)"("Format"=w164) -> ()  [unwired: 2 in, 2 out]
        n109 = call "Results FGV.vi"("Function"=enum16{"write", "read"}."write", "Input Signals"=w179) -> ()  [unwired: 4 in, 2 out]
        "Waveform Graph" <- w150
      }
      frame 4 {
        # "This code stops the AI/AO Tasks, erases them, and ends program execution."
        n110 = local read "simulate?"() -> (w232:bool)
        n111 = case shown="False" w232 {
          frame False {
            n112 = disable-structure shown="Default" {
              frame condition #0 (active) {
                n113 = local read "AO Task"() -> (w236:refnum<k21>[])
                n114 = local read "AI task"() -> (w237:refnum<k21>[])
                n115 = flat-sequence {
                  tunnel: w237 -> [w245]
                  tunnel: [w244] -> w242
                  tunnel: w236 -> [w244]
                  tunnel: [w243] -> w241
                  tunnel: w242 -> [w251]
                  tunnel: w241 -> [w250]
                  tunnel: [w250] -> w240
                  tunnel: [w249] -> w239
                  tunnel: w240 -> [w255]
                  tunnel: w239 -> [w256]
                  tunnel: [w256] -> w238
                  tunnel: w238 -> [w259]
                  frame #0 {
                    n116 = for {
                      tunnel: w245 -> [w248] mode=indexing
                      tunnel: [w246] -> w243 mode=indexing
                      n117 = call <vilib>:"DAQmx Stop Task.vi"("task/channels in"=w248) -> ("task out"=w246:refnum<k21>)  [unwired: 13 in, 1 out]
                      n118 = Wait (ms)(milliseconds to wait=u32 50) -> ()  [unwired: 1 out]
                    }
                  }
                  frame #1 {
                    n119 = for {
                      tunnel: w251 -> [w254] mode=indexing
                      tunnel: [w252] -> w249 mode=indexing
                      n120 = call <vilib>:"DAQmx Stop Task.vi"("task/channels in"=w254) -> ("task out"=w252:refnum<k21>)  [unwired: 13 in, 1 out]
                      n121 = Wait (ms)(milliseconds to wait=u32 50) -> ()  [unwired: 1 out]
                    }
                  }
                  frame #2 {
                    n122 = for {
                      tunnel: w255 -> [w258] mode=indexing
                      n123 = call <vilib>:"DAQmx Clear Task.vi"("task in"=w258) -> ()  [unwired: 14 in, 1 out]
                      n124 = Wait (ms)(milliseconds to wait=u32 50) -> ()  [unwired: 1 out]
                    }
                  }
                  frame #3 {
                    n125 = for {
                      tunnel: w259 -> [w261] mode=indexing
                      n126 = call <vilib>:"DAQmx Clear Task.vi"("task in"=w261) -> ()  [unwired: 14 in, 1 out]
                      n127 = Wait (ms)(milliseconds to wait=u32 50) -> ()  [unwired: 1 out]
                    }
                  }
                }
              }
              frame condition #1 {
              }
            }
          }
          frame True {
          }
        }
      }
      frame 5 {
        # "This code stops AI/AO tasks, deletes them, and restarts program execution."
        n128 = local read "simulate?"() -> (w263:bool)
        n129 = case shown="False" w263 {
          frame False {
            n130 = disable-structure shown="Default" {
              frame condition #0 (active) {
                n131 = local read "AO Task"() -> (w267:refnum<k21>[])
                n132 = local read "AI task"() -> (w268:refnum<k21>[])
                n133 = flat-sequence {
                  tunnel: w268 -> [w276]
                  tunnel: [w275] -> w273
                  tunnel: w267 -> [w275]
                  tunnel: [w274] -> w272
                  tunnel: w273 -> [w282]
                  tunnel: w272 -> [w281]
                  tunnel: [w281] -> w271
                  tunnel: [w280] -> w270
                  tunnel: w271 -> [w286]
                  tunnel: w270 -> [w287]
                  tunnel: [w287] -> w269
                  tunnel: w269 -> [w290]
                  frame #0 {
                    n134 = for {
                      tunnel: w276 -> [w279] mode=indexing
                      tunnel: [w277] -> w274 mode=indexing
                      n135 = call <vilib>:"DAQmx Stop Task.vi"("task/channels in"=w279) -> ("task out"=w277:refnum<k21>)  [unwired: 13 in, 1 out]
                      n136 = Wait (ms)(milliseconds to wait=u32 50) -> ()  [unwired: 1 out]
                    }
                  }
                  frame #1 {
                    n137 = for {
                      tunnel: w282 -> [w285] mode=indexing
                      tunnel: [w283] -> w280 mode=indexing
                      n138 = call <vilib>:"DAQmx Stop Task.vi"("task/channels in"=w285) -> ("task out"=w283:refnum<k21>)  [unwired: 13 in, 1 out]
                      n139 = Wait (ms)(milliseconds to wait=u32 50) -> ()  [unwired: 1 out]
                    }
                  }
                  frame #2 {
                    n140 = for {
                      tunnel: w286 -> [w289] mode=indexing
                      n141 = call <vilib>:"DAQmx Clear Task.vi"("task in"=w289) -> ()  [unwired: 14 in, 1 out]
                      n142 = Wait (ms)(milliseconds to wait=u32 50) -> ()  [unwired: 1 out]
                    }
                  }
                  frame #3 {
                    n143 = for {
                      tunnel: w290 -> [w292] mode=indexing
                      n144 = call <vilib>:"DAQmx Clear Task.vi"("task in"=w292) -> ()  [unwired: 14 in, 1 out]
                      n145 = Wait (ms)(milliseconds to wait=u32 50) -> ()  [unwired: 1 out]
                    }
                  }
                }
              }
              frame condition #1 {
              }
            }
          }
          frame True {
          }
        }
      }
    }
  }
